vi "2num.vi"() -> ()   [LabVIEW 2019]
uses:
  <vilib>/ErrorRing/Error Ring.xnode
  my_state_machine/control.ctl
panel:
  in  "stop":bool
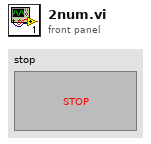
[diagram p1: front panel]
types:
  T1 = typedef "control.ctl" = enum16{""}
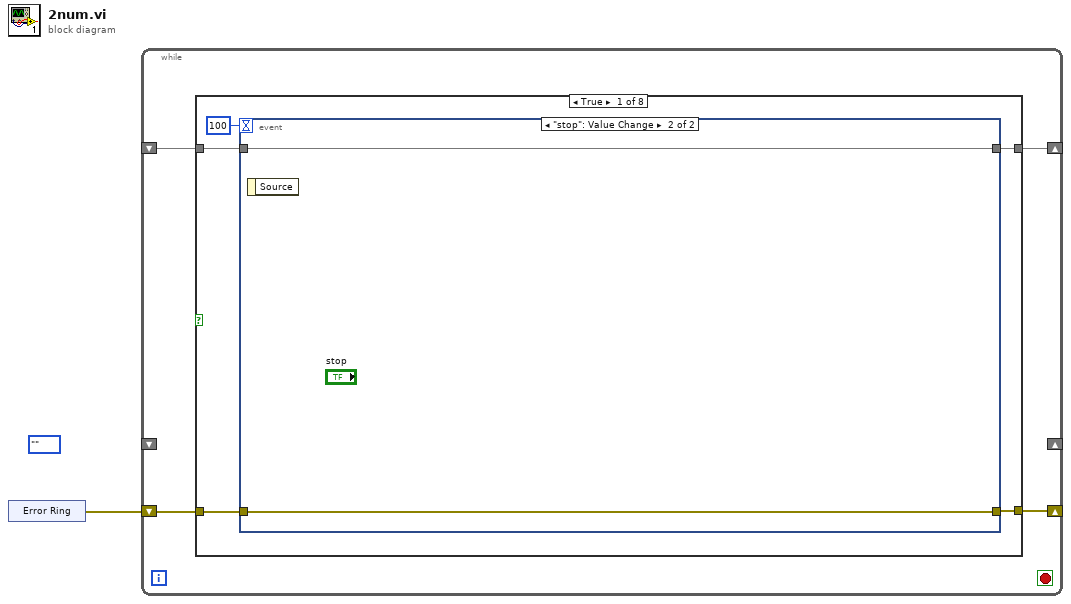
[diagram p0: block diagram]
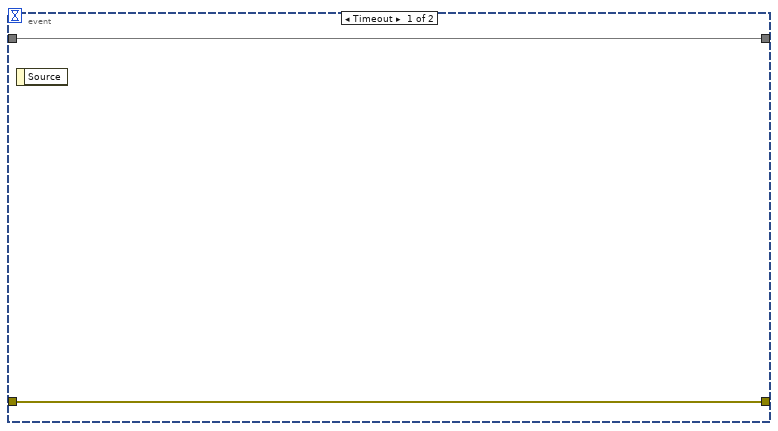
[diagram p2: hidden frame]
diagram:
  (unwired) control.""
  n1 = xnode "Error Ring"() -> ("error out"=w1:errorcluster)
  n2 = while {
    shift-right: [w2] -> _
    shift-left: _ -> [w3]
    shift-right: _ -> [_]
    shift-left: _ -> [_]
    shift-right: [w4] -> _
    shift-left: w1 -> [w5]
    stop <- _ stop-if-true
    n3 = case shown="\"idle\"" {
      selector: _ -> [_ _ _ _ _ _ _ _]
      tunnel: w5 -> [w10 _ _ _ _ _ _ _]
      tunnel: [w9 _ _ _ _ _ _ _] -> w4
      tunnel: w3 -> [w7 w15 w16 w17 w18 w19 w20 w21]
      tunnel: [w6 w15 w16 w17 w18 w19 w20 w21] -> w2
      frame True {
        n4 = event shown="[1] \"stop\": Value Change" {
          selector: _ -> [_ _]
          dyn-events: _ -> [_ _]
          timeout: 100 -> [_ _]
          tunnel: w10 -> [w12 w14]
          tunnel: [w12 w14] -> w9
          tunnel: w7 -> [w11 w13]
          tunnel: [w11 w13] -> w6
          event Timeout {
            n5 = event-data() -> ()  [unwired: 1 in, 1 out]
          }
          event "stop": Value Change {
            n6 = event-data() -> ()  [unwired: 1 in, 1 out]
          }
        }
      }
      frame False {
      }
      frame True {
      }
      frame True {
      }
      frame True {
      }
      frame True {
      }
      frame True {
      }
      frame True {
      }
    }
  }
